vi "Add Response - Byte Count.vi"(8 "error in (no error)":errorcluster, 10 "Settings":T1 {"Channel Refnum" format="%.0x"; "Linked Channels"."Channel Refnum" format="%.0x"}, 11 "Message in":T3 format="%.0x") -> (0 "error out":errorcluster, 3 "Message out":T3 format="%.0x")   [LabVIEW 2018, in "Instrument Addon Scripting API.lvlib"]
doc: "Adds or creates (if it does not already exists) a Response section to the specified Message. If the provided NodeID does not correspond to an existing Message section, this VI will throw an error. \n\nIf you want to use \"Linked Channels\" with the \"Response Format\" string, make sure that the Channel Refnums used in the \"Linked Channels\" parameter already exist before calling this SubVI.\n\nNotes: \n- This VI will throw an error if the \"Response Format\" string contains duplicate variable names\n- This VI will throw an error if the number of variables in the \"Response Format\" string is different from the number of linked channels \n- This VI will throw an error if the variable names in the \"Response Format\" string does not correspond to the variable names used in the \"Linked Channels\" parameter."
uses:
  Instrument Addon Scripting API.lvlib
  <vilib>/NI Veristand/Custom Device API/Custom Device Item Ref.ctl
  TypeDefs/ByteCount Response Settings.ctl
  TypeDefs/Linked Channel.ctl
  Addon/Addon Shared/Types/FG Control.ctl
  Addon/Addon Shared/Types/Response Parameters.ctl
  Addon/Addon Shared/Types/Linked Channel Cluster.ctl
  Addon/Addon Shared/Types/Response Wait Type.ctl
  Addon/Addon Shared/SubVIs/Constants.vi
  <vilib>/NI/NI VeriStand Advanced SysDef API/_SubVIs/SysDef.Search.GUID.vi
  <vilib>/NI Veristand/Custom Device API/NI VeriStand - Get Item Property.vi
  <vilib>/NI Veristand/Custom Device API/Get Item Property (String).vi
  <vilib>/NI Veristand/Custom Device API/Get Item Property (String Array).vi
  <vilib>/NI Veristand/Custom Device API/Get Item Property (Double).vi
  <vilib>/NI Veristand/Custom Device API/Get Item Property (U32).vi
  <vilib>/NI Veristand/Custom Device API/Get Item Property (Boolean).vi
  <vilib>/NI Veristand/Custom Device API/NI VeriStand - Set Item Property.vi
  <vilib>/NI Veristand/Custom Device API/Set Item Property (String).vi
  <vilib>/NI Veristand/Custom Device API/Set Item Property (String Array).vi
  <vilib>/NI Veristand/Custom Device API/Set Item Property (Double).vi
  <vilib>/NI Veristand/Custom Device API/Set Item Property (U32).vi
  <vilib>/NI Veristand/Custom Device API/Set Item Property (Boolean).vi
  <vilib>/NI/NI VeriStand Advanced SysDef API/SysDef API/Advanced System Definition.lvlib
  Addon/Addon Shared/Instrument Addon Shared.lvlib
  <vilib>/NI Veristand/Custom Device API/Custom Device API.lvlib
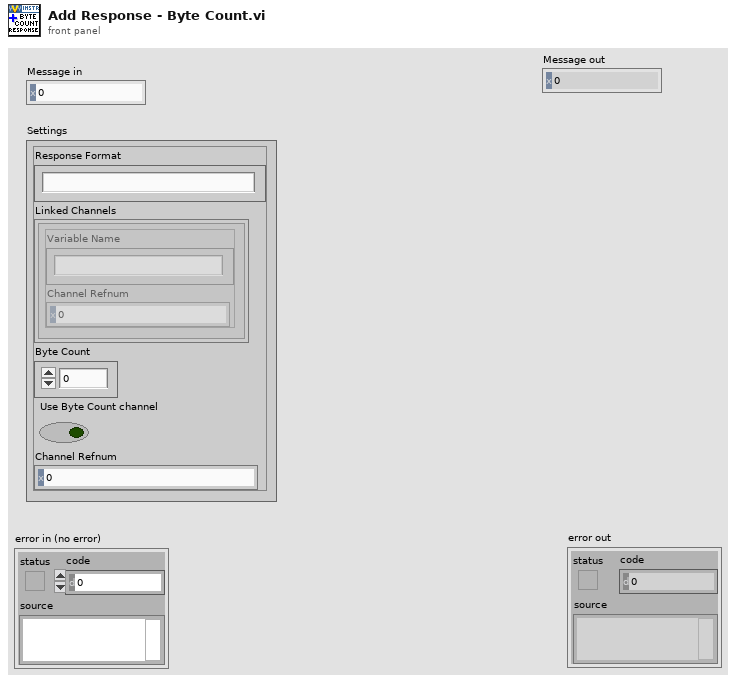
[diagram p1: front panel]
types:
  T1 = typedef "Instrument Addon Scripting API.lvlib/ByteCount Response Settings.ctl" = cluster{"Response Format":string, "Linked Channels":T2[], "Byte Count":i32, "Use Byte Count channel":bool, "Channel Refnum":T3}
  T2 = typedef "Instrument Addon Scripting API.lvlib/Linked Channel.ctl" = cluster{"Variable Name":string, "Channel Refnum":T3}
  T3 = typedef "Custom Device API.lvlib/Custom Device Item Ref.ctl" = u64
  T4 = typedef "Instrument Addon Shared.lvlib/Response Wait Type.ctl" = enum16{"Byte Count", "Wait sec"}
  T5 = typedef "Instrument Addon Shared.lvlib/Response Parameters.ctl" = cluster{"Response":string, "Linked Channels":T6[], "Type Value":dbl, "Wait Type":T4, "Use Channel":bool, "Channel Path":string}
  T6 = typedef "Instrument Addon Shared.lvlib/Linked Channel Cluster.ctl" = cluster{"Variable Name":string, "GUID":string}
  T7 = typedef "Instrument Addon Shared.lvlib/FG Control.ctl" = enum16{"Get", "Set"}
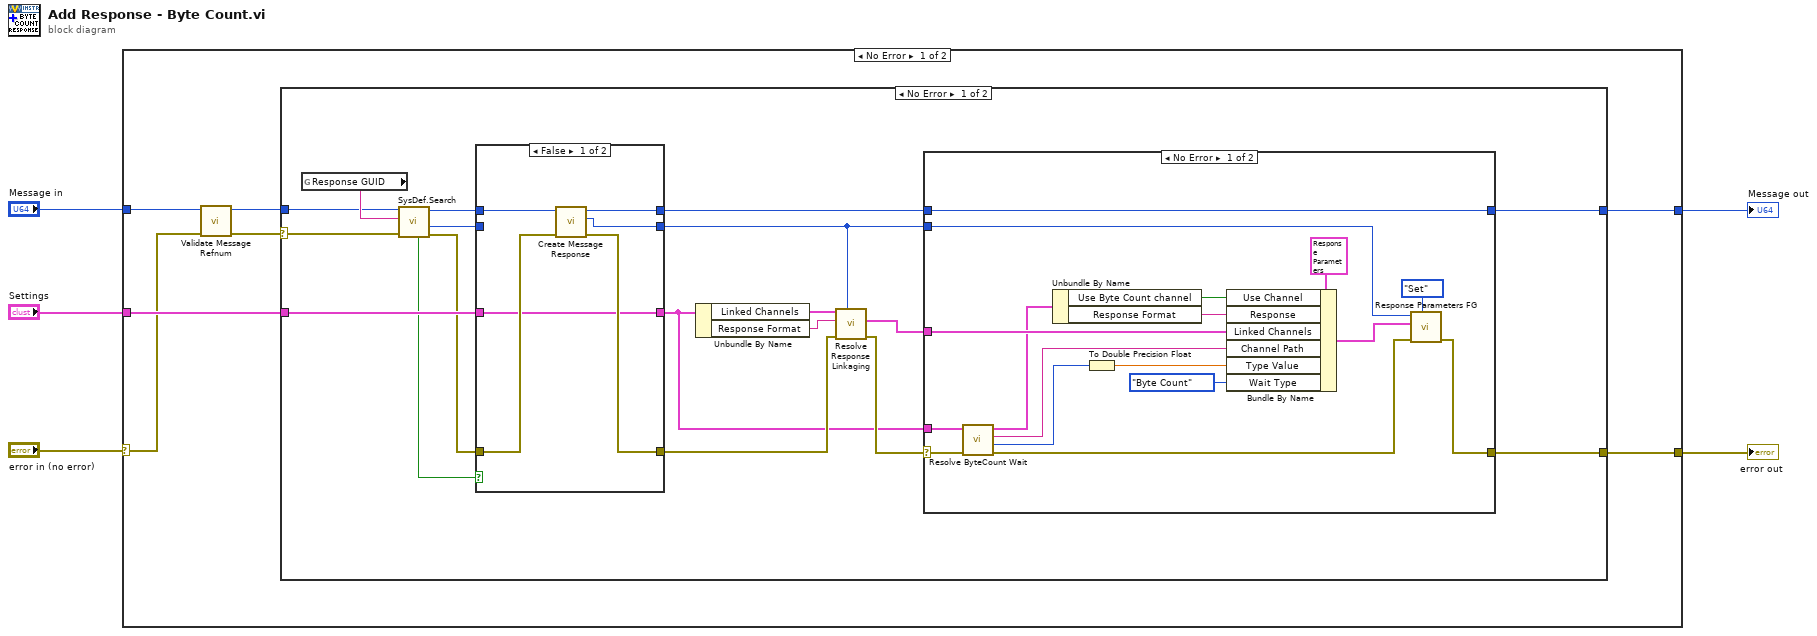
[diagram p0: block diagram]
diagram:
  n1 = case shown="No Error" "error in (no error)" {
    selector: "error in (no error)" -> [w7 w62]
    tunnel: "Message in" -> [w9 w63]
    tunnel: "Settings" -> [w12 _]
    tunnel: [w11 w63] -> w2
    tunnel: [w10 w62] -> w1
    frame No Error {
      n2 = call "Validate Message Refnum.vi"("error in (no error)"=w7, "Message in"=w9) -> ("error out"=w6:errorcluster, "Item Ref out"=w8:T3)  [unwired: 8 in]
      n3 = case shown="No Error" w6 {
        selector: w6 -> [w13 w60]
        tunnel: w12 -> [w30 _]
        tunnel: [w29 w61] -> w11
        tunnel: [w28 w60] -> w10
        tunnel: w8 -> [w14 w61]
        frame No Error {
          n4 = global read "Constants.vi" "Response GUID"() -> (w27:string)
          n5 = call-poly <vilib>:"SysDef.Search.vi"("error in (no error)"=w13, "GUID"=w27, "nodeID"=w14) -> ("error out"=w24:errorcluster, "Value out"=w18:u64, "nodeID out"=w25:u64, "Found?"=w26:bool)  [unwired: 5 in]
          n6 = case shown="False" w26 {
            tunnel: w18 -> [_ w59]
            tunnel: w25 -> [w55 w57]
            tunnel: w24 -> [w54 w58]
            tunnel: [w53 w58] -> w23
            tunnel: [w52 w59] -> w20
            tunnel: [w51 w56] -> w15
            tunnel: w30 -> [w51 w56]
            tunnel: [w50 w57] -> w19
            frame False {
              n7 = call "Create Message Response.vi"("error in (no error)"=w54, "Message in"=w55) -> ("error out"=w53:errorcluster, "Response Section Ptr"=w52:T3, "Message out"=w50:T3)  [unwired: 7 in]
            }
            frame True {
            }
          }
          n8 = Unbundle By Name(w15) -> ("Linked Channels"=w17:T2[], "Response Format"=w16:string)
          n9 = call "Resolve Response Linkaging.vi"("Response Refnum in"=w20, "error in (no error)"=w23, "Response Format"=w16, "Linked Channels"=w17) -> ("error out"=w22:errorcluster, "Linked Channels out"=w21:T6[])  [unwired: 6 in]
          n10 = case shown="No Error" w22 {
            selector: w22 -> [w35 w48]
            tunnel: w21 -> [w43 _]
            tunnel: [w42 w48] -> w28
            tunnel: w20 -> [w39 _]
            tunnel: w19 -> [w38 w49]
            tunnel: [w38 w49] -> w29
            tunnel: w15 -> [w36 _]
            frame No Error {
              n11 = call "Resolve ByteCount Wait .vi"("error in (no error)"=w35, "Settings in"=w36) -> ("error out"=w34:errorcluster, "Byte Count"=w33:i32, "Channel Path"=w32:string, "Settings out"=w31:T1)  [unwired: 6 in]
              n12 = Unbundle By Name(w31) -> ("Use Byte Count channel"=w37:bool, "Response Format"=w45:string)
              n13 = To Double Precision Float(number=w33) -> (double precision float=w41:dbl)
              n14 = Bundle By Name(cluster=T5 {"Response"="", "Linked Channels"=[], "Type Value"=1.0, "Wait Type"=enum."Wait sec", "Use Channel"=FALSE, "Channel Path"=""} ("Reponse Parameters"), "Use Channel"=w37, "Response"=w45, "Linked Channels"=w43, "Channel Path"=w32, "Type Value"=w41, "Wait Type"=Response_Wait_Type."Byte Count") -> (w44:T5)
              n15 = call "Response Parameters FG.vi"("Action"=FG_Control."Set", "error in (no error)"=w34, "Reponse Parameters"=w44, "Item Ref in"=w39) -> ("error out"=w42:errorcluster)  [unwired: 5 in, 2 out]
            }
            frame Error {
            }
          }
        }
        frame Error {
        }
      }
    }
    frame Error {
    }
  }
  "error out" <- w1
  "Message out" <- w2
